vi "loadDataNodeEnd.vi"(8 "error in (no error)":errorcluster, 10 "XML Refnum in":refnum<file>, 11 "Parameter in":refnum<class "Parameter.lvclass">) -> (0 "error out":errorcluster, 2 "XML Refnum out":refnum<file>, 3 "Parameter out":refnum<class "Parameter.lvclass">)   [LabVIEW 2013, in "Parameter.lvclass"]
doc: "Part of the file loading process. Occurs at the end of a node being loaded. Includes checking the end of the tag which has the format </tag>."
uses:
  Parameter.lvclass
  xCE/xceNode/xceNode.lvclass
  XML Parser/XML Parser.lvclass
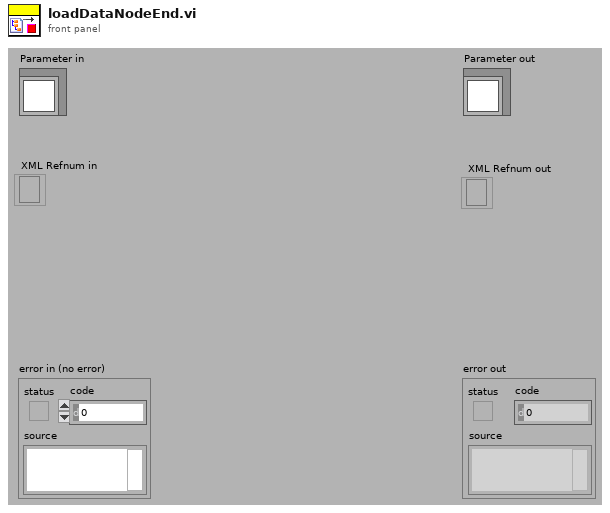
[diagram p1: front panel]
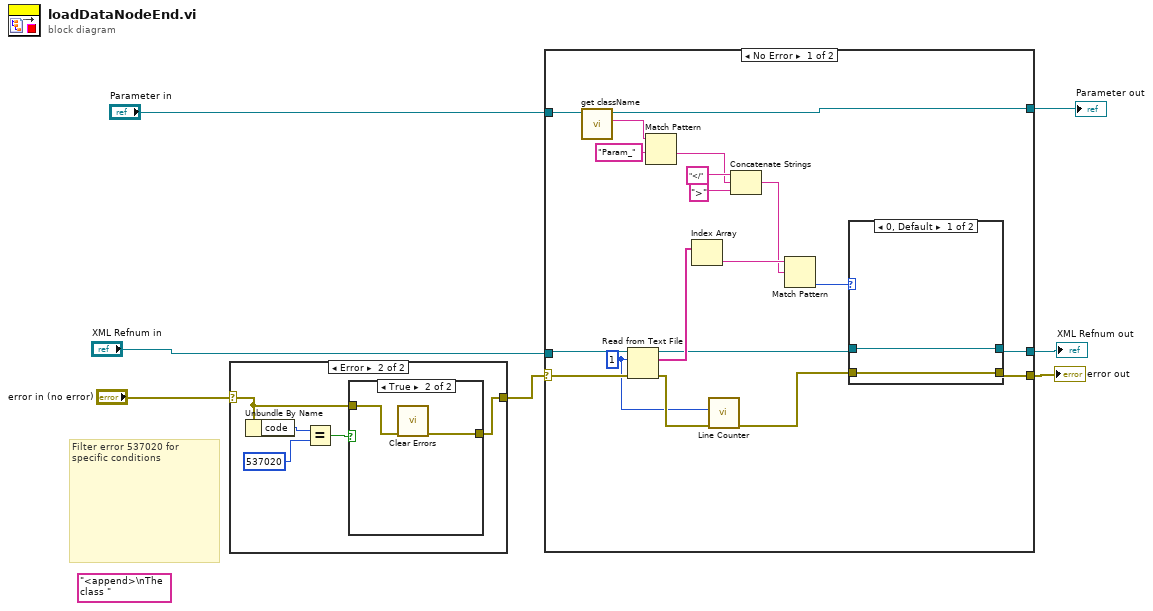
[diagram p0: block diagram]
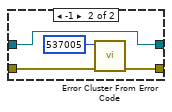
[diagram p4: hidden frame]
diagram:
  (unwired) "<append>\nThe class " ("source")
  # "Filter error 537020 for specific conditions"
  n1 = case shown="Error" "error in (no error)" {
    selector: "error in (no error)" -> [w8 w10]
    tunnel: [w8 w9] -> w1
    frame No Error {
    }
    frame Error {
      n2 = Unbundle By Name(w10) -> ("code"=w13:i32)
      n3 = Equal?(x=w13, y=537020) -> (x = y?=w11:bool)
      n4 = case shown="True" w11 {
        tunnel: w10 -> [w14 w16]
        tunnel: [w14 w15] -> w9
        frame False {
        }
        frame True {
          n5 = call <vilib>:"Clear Errors.vi"("error in (no error)"=w16) -> ("error out"=w15:errorcluster)  [unwired: 6 in]
        }
      }
    }
  }
  n6 = case shown="No Error" w1 {
    selector: w1 -> [w35 w44]
    tunnel: [w27 w44] -> w5
    tunnel: [w33 w42] -> w4
    tunnel: "XML Refnum in" -> [w34 w43]
    tunnel: [w25 w43] -> w6
    tunnel: "Parameter in" -> [w23 w42]
    frame No Error {
      w17 = 1 ("count")
      n7 = call "get className.vi"("xceNode in"=w23) -> ("Class name"=w21:string, "xceNode out"=w33:refnum<class "Parameter.lvclass">)  [unwired: 8 in, 1 out]
      n8 = Read from Text File(file (use dialog)=w34, count=w17, error in=w35) -> (refnum out=w26:refnum<file>, text=w30:string[], error out=w19:errorcluster)  [unwired: 1 in, 1 out]
      n9 = Match Pattern(string=w21, regular expression="Param_") -> (after substring=w20:string)  [unwired: 1 in, 3 out]
      n10 = Index Array(array=w30) -> (element=w29:string)  [unwired: 1 in]
      n11 = call "Line Counter.vi"("error in (no error)"=w19, "# of lines to increment (1)"=w17) -> ("error out"=w18:errorcluster)  [unwired: 8 in, 1 out]
      n12 = Concatenate Strings("</", w20, ">") -> (w22:string)
      n13 = Match Pattern(string=w29, regular expression=w22) -> (offset past match=w28:i32)  [unwired: 1 in, 3 out]
      n14 = case shown="0, Default" w28 {
        tunnel: w18 -> [w37 w41]
        tunnel: [w37 w39] -> w27
        tunnel: w26 -> [w36 w38]
        tunnel: [w36 w38] -> w25
        frame 0, Default {
        }
        frame -1 {
          n15 = call <vilib>:"Error Cluster From Error Code.vi"("error in (no error)"=w41, "error code (0)"=537005) -> ("error out"=w39:errorcluster)  [unwired: 7 in]
        }
      }
    }
    frame Error {
    }
  }
  "error out" <- w5
  "Parameter out" <- w4
  "XML Refnum out" <- w6
